vi "View.vi"(8 "error in (no error)":errorcluster, 10 "Debugger":refnum<class "Debug Process.lvclass">, 11 "List View In":refnum<class "Variant View.lvclass">) -> (0 "error out":errorcluster)   [LabVIEW 2020, in "Variant View.lvclass"]
uses:
  Variant View.lvclass
  C:/Users/anton/Documents/GitHub/triarc-debugger/source/Debug View/Debug View.lvclass
  Process/Debug Process.lvclass
  Process/Debug Process.lvclass/Debug Process.ctl
  Debug View/Debug View.lvclass/Debug View.ctl
  Variant View.lvclass/Variant View.ctl
  Debugger/Debugger.lvclass
  Debug Data/Debug Data.lvclass/Debug Data.ctl
  Variant View Model/Variant View Model.lvclass
  Debug View/Debug View.lvclass
  Debug Data/Debug Data.lvclass
panel:
  in  "Variant":variant caption="Message data"
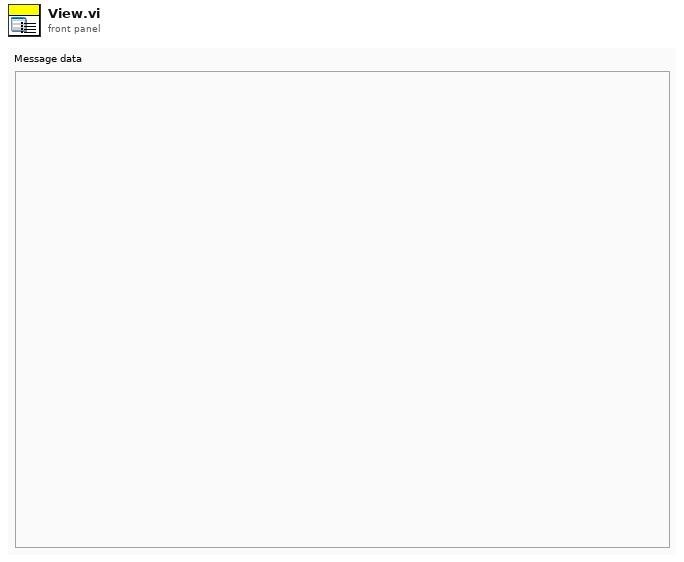
[diagram p1: front panel]
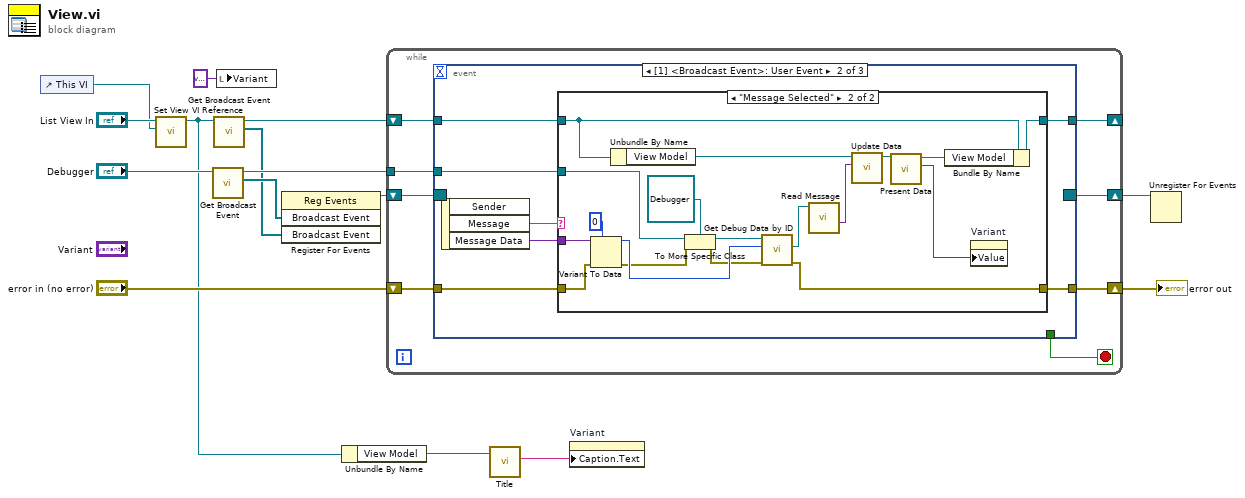
[diagram p0: block diagram]
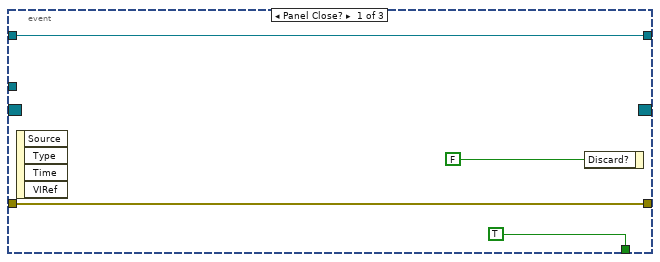
[diagram p2: hidden frame]
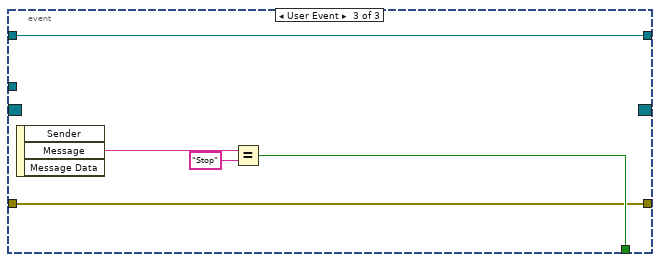
[diagram p4: hidden frame]
diagram:
  n1 = control-ref of="This VI"() -> (w2:refnum<vi>)
  n2 = call "Set View VI Reference.vi"("View VI ref"=w2, "Debug View in"="List View In") -> ("Debug View out"=w3:refnum<class "Variant View.lvclass">)  [unwired: 8 in, 1 out]
  n3 = call "Get Broadcast Event.vi"("Process in"="Debugger") -> ("Broadcast Event"=w7:refnum<user-event>[], "Process out"=w9:refnum<class "Debug Process.lvclass">)  [unwired: 8 in, 1 out]
  n4 = call "Get Broadcast Event.vi"("Debug View In"=w3) -> ("Broadcast Event"=w4:refnum<user-event>[], "Debug View Out"=w5:refnum<class "Variant View.lvclass">)  [unwired: 8 in, 1 out]
  n5 = local write "Variant"(variant ("Variant")) -> ()
  n6 = register-events(w7, w4) -> (reference out=w8:refnum<event-registration>)  [unwired: 2 in, 1 out]
  n7 = Unbundle By Name(w3) -> ("View Model"=w12:refnum<class "Variant View Model.lvclass">)
  n8 = while {
    shift-right: [w22] -> _
    shift-left: w5 -> [w23]
    shift-right: [w21] -> w15
    shift-left: "error in (no error)" -> [w20]
    shift-right: [w19] -> w13
    shift-left: w8 -> [w18]
    tunnel: w9 -> [w17]
    stop <- w16 stop-if-true
    n9 = event shown="[1] <Broadcast Event>: User Event" {
      selector: w18 -> [_ _ _]
      dyn-events: [_ _ _] -> w19
      timeout: _ -> [_ _ _]
      tunnel: w23 -> [w27 w30 w55]
      tunnel: [w27 w29 w55] -> w22
      tunnel: [w26 w33 w56] -> w21
      tunnel: w20 -> [w26 w32 w56]
      tunnel: w17 -> [_ w28 _]
      tunnel: [TRUE ("Discard?") _ w57] -> w16
      event Panel Close? {
        n10 = event-data() -> ()  [unwired: 1 in, 4 out]
        n11 = event-data("Discard?"=FALSE) -> ()  [unwired: 1 in, 1 out]
      }
      event User Event {
        n12 = event-data() -> ("Message"=w34:string, "Message Data"=w31:variant)  [unwired: 1 in, 1 out]
        n13 = case shown="\"Message Selected\"" w34 {
          tunnel: [w36 w37] -> w33
          tunnel: w32 -> [w36 w46]
          tunnel: w31 -> [_ w48]
          tunnel: w30 -> [w35 w54]
          tunnel: [w35 w51] -> w29
          tunnel: w28 -> [_ w45]
          frame Default {
          }
          frame "Message Selected" {
            n14 = Variant To Data(error in=w46, type=u32 0 ("Message ID"), Variant=w48) -> (data=w42:u32, error out=w40:errorcluster)
            n15 = Unbundle By Name(w54) -> ("View Model"=w53:refnum<class "Variant View Model.lvclass">)
            n16 = To More Specific Class(target class=refnum<class "Debugger.lvclass"> refnum ("Debugger out"), reference=w45, error in=w40) -> (specific class reference=w44:refnum<class "Debugger.lvclass">, error out=w41:errorcluster)
            n17 = call "Get Debug Data by ID.vi"("error in (no error)"=w41, "Message ID"=w42, "Debugger In"=w44) -> ("error out"=w37:errorcluster, "Debug Data"=w39:refnum<class "Debug Data.lvclass">)  [unwired: 6 in, 1 out]
            n18 = call "Read Message.vi"("Debug Data in"=w39) -> ("Message Data"=w38:variant)  [unwired: 8 in, 2 out]
            n19 = call-dynamic "Update Data.vi"("Message Data"=w38, "List Seen Processes View Model In"=w53) -> ("List Seen Processes View Model Out"=w49:refnum<class "Variant View Model.lvclass">)  [unwired: 8 in, 1 out]
            n20 = call "Present Data.vi"("List Seen Processes View Model In"=w49) -> ("Message Data"=w52:variant, "List Seen Processes View Model Out"=w50:refnum<class "Variant View Model.lvclass">)  [unwired: 8 in, 1 out]
            n21 = Bundle By Name(cluster=w54, "View Model"=w50) -> (w51:refnum<class "Variant View.lvclass">)
            n22 = property on="Variant" class="LVVar"("Value"=w52) -> ()  [unwired: 2 in, 2 out]
          }
        }
      }
      event User Event {
        n23 = event-data() -> ("Message"=w59:string)  [unwired: 1 in, 2 out]
        n24 = Equal?(x=w59, y="Stop") -> (x = y?=w57:bool)
      }
    }
  }
  "error out" <- w15
  n25 = call-dynamic "Title.vi"("List Box View Model in"=w12) -> ("Title"=w11:string)  [unwired: 8 in, 2 out]
  n26 = property on="Variant" class="LVVar"("Caption.Text"=w11) -> ()  [unwired: 2 in, 2 out]
  n27 = Unregister For Events(event registration refnum=w13) -> ()  [unwired: 1 in, 1 out]
